vi "Find Contours.vi"(5 "Contour Approximation Mode (Default: SIMPLE)":T5=enum."SIMPLE", 7 "Contour Retrieval Modes (Default: TREE)":T4=enum."TREE", 8 "error in (no error)":errorcluster, 11 "Greyscale Image":T6) -> (0 "error out":errorcluster, 2 "Found Contours":T1[](array[typedef]), 3 "Greyscale Image (Duplicate)":T6)   [LabVIEW 2020, in "g_ar_toolkit.feature_detection.lvlib"]
uses:
  g_ar_toolkit.feature_detection.lvlib
  g_ar_toolkit.image/Greyscale Image.ctl
  Contour Approximation Mode.ctl
  Contour Retrieval Modes.ctl
  Found Contour.ctl
  g_ar_toolkit.common/Image Point (Integer).ctl
  Contour Hierarchy.ctl
  g_ar_toolkit.common/g_ar_toolkit.common.lvlib
  g_ar_toolkit.image/g_ar_toolkit.image.lvlib
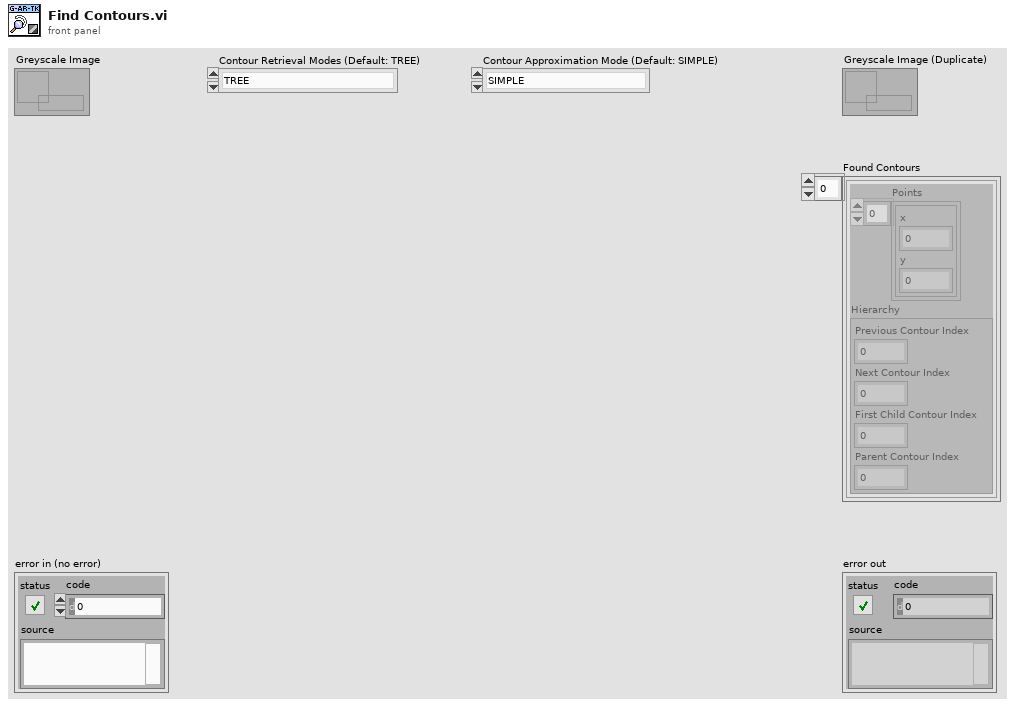
[diagram p1: front panel]
types:
  T1 = typedef "g_ar_toolkit.feature_detection.lvlib/Found Contour.ctl" = cluster{"Points":T2[], "Hierarchy":T3}
  T2 = typedef "g_ar_toolkit.common.lvlib/Image Point (Integer).ctl" = cluster{"x":i32, "y":i32}
  T3 = typedef "g_ar_toolkit.feature_detection.lvlib/Contour Hierarchy.ctl" = cluster{"Previous Contour Index":i32, "Next Contour Index":i32, "First Child Contour Index":i32, "Parent Contour Index":i32}
  T4 = typedef "g_ar_toolkit.feature_detection.lvlib/Contour Retrieval Modes.ctl" = enum16{"EXTERNAL", "LIST", "CCOMP", "TREE"}
  T5 = typedef "g_ar_toolkit.feature_detection.lvlib/Contour Approximation Mode.ctl" = enum16{"NONE", "SIMPLE", "TC89_L1", "TC89_KCOS"}
  T6 = typedef "g_ar_toolkit.image.lvlib/Greyscale Image.ctl" = refnum<data-value>
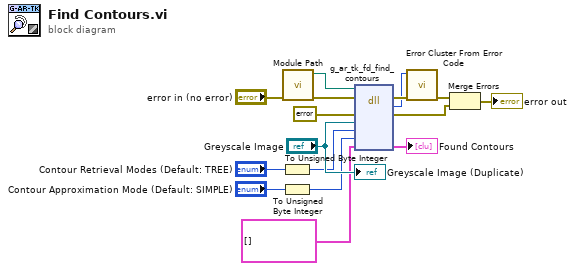
[diagram p0: block diagram]
diagram:
  n1 = To Unsigned Byte Integer(number="Contour Retrieval Modes (Default: TREE)") -> (unsigned 8bit integer=w5:u8)
  n2 = To Unsigned Byte Integer(number="Contour Approximation Mode (Default: SIMPLE)") -> (unsigned 8bit integer=w4:u8)
  n3 = call "Module Path.vi"("error in (no error)"="error in (no error)") -> ("error out"=w2:errorcluster, "Path"=w1:path)  [unwired: 9 in]
  n4 = dll-call lib="?" fn="g_ar_tk_fd_find_contours" ("g_ar_toolkit.*.*:g_ar_tk_image_draw_line")(path in=w1, error in=w2, "error_cluster"=errorcluster {"status"=FALSE, "code"=0, "source"=""} ("error constant"), "EDVR src"="Greyscale Image", "retrieval_mode"=w5, "contour_mode"=w4, "contours"=T1[] [] ("Array")) -> (error out=w13:errorcluster, "MgErr"=w12:i32, "error_cluster"=w9:errorcluster, "contours"=→"Found Contours":T1[])  [unwired: 4 in, 1 out]
  n5 = call <vilib>:"Error Cluster From Error Code.vi"("error in (no error)"=w13, "error code (0)"=w12) -> ("error out"=w11:errorcluster)  [unwired: 7 in]
  n6 = Merge Errors(w11, w9) -> (→"error out":errorcluster)
  "Greyscale Image (Duplicate)" <- "Greyscale Image"
